vi "rgb to grayscale pixel.vi"(7 "Color (U32)":u32) -> (8 "Grayscale (U8)":u8)   [LabVIEW 2018]
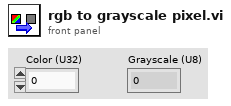
[diagram p1: front panel]
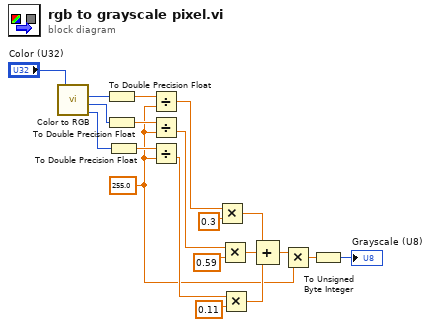
[diagram p0: block diagram]
diagram:
  w2 = 255.0 ("y")
  n1 = call <vilib>:"Color to RGB.vi"("Color"="Color (U32)") -> ("R"=w17:u8, "G"=w18:u8, "B"=w19:u8)  [unwired: 1 out]
  n2 = To Double Precision Float(number=w17) -> (double precision float=w15:dbl)
  n3 = To Double Precision Float(number=w18) -> (double precision float=w14:dbl)
  n4 = To Double Precision Float(number=w19) -> (double precision float=w13:dbl)
  n5 = Divide(x=w15, y=w2) -> (x/y=w11:dbl)
  n6 = Divide(x=w14, y=w2) -> (x/y=w10:dbl)
  n7 = Divide(x=w13, y=w2) -> (x/y=w8:dbl)
  n8 = Multiply(x=w11, y=0.3) -> (x*y=w6:dbl)
  n9 = Multiply(x=w10, y=0.59) -> (x*y=w5:dbl)
  n10 = Multiply(x=w8, y=0.11) -> (x*y=w4:dbl)
  n11 = Compound Arithmetic op=ADD(w6, w5, w4) -> (w3:dbl)
  n12 = Multiply(x=w3, y=w2) -> (x*y=w1:dbl)
  n13 = To Unsigned Byte Integer(number=w1) -> (unsigned 8bit integer=→"Grayscale (U8)":u8)
